vi "Gray's Mod Motor Controler.vi"() -> ()   [LabVIEW 2009]
uses:
  <vilib>/eio/EIONode/EIONode.xnode
  <vilib>/rvi/eio/nirviEIOImplementation/nirviEIOImplementation.xnode
  <vilib>/rvi/eio/common/nirviEmuTemplateMethod_noerrors.vi
  <vilib>/rvi/eio/common/nirviEmuClasses.ctl
  <vilib>/Platform/TimedLoop/XDataNode/XDataNode.xnode
  <vilib>/Platform/TimedLoop/XDataNode/loadlvalarms.vi
  <vilib>/Platform/TimedLoop/XDataNode/timing_clust.ctl
  <vilib>/Platform/TimedLoop/XDataNode/nitl_modes.ctl
  <vilib>/Platform/TimedLoop/XDataNode/wakeup.ctl
  <vilib>/Platform/TimedLoop/XDataNode/XDNodeRunTimeDep.lvlib
panel:
  in  "Steering Encoder Reset \nPosition Whole Rotations":i32
  in  "Counts per Drive Position 2":i32=205386
  in  "Drive Encoder Reset \nPosition Fractional":i32
  in  "Counts per Drive Position":i32=205386
  in  "Stop":bool=TRUE
  out "Drive Motor Speed (cpt)":fxp<+/-,20,1>
  out "Drive Encoder Delta (ticks)":u32
  in  "Drive Motor Speed Setpoint (mph)":fxp<+/-,20,7>
  in  "Drive Speed Proportional Control Feedback Gain":fxp<+/-,20,5>
  out "Drive Motor Speed (Volts)":fxp<+/-,20,5> format="%.17g"
  in  "Drive Conversion: \nmph to counts per tick":fxp<+/-,20,0>
  in  "Drive Encoder Offset":fxp<+/-,20,1>
  in  "Steering Proportional Control Feedback Gain":i32
  in  "Steer Motor Setpoint (degrees)":i8
  in  "Steering Encoder Offset from 0 counts":i32
  in  "Steering Conversion: degrees to ticks":i32
  out "Steering Motor Speed (Volts)":fxp<+/-,20,5> format="%.17g"
  out "Steering Position":i32
  out "Steering Encoder Index":i32
  out "Steering Encoder Raw":i32
  in  "Steering Encoder Reset":bool
  in  "Steering Encoder Reset \nPositions Fractional":i32
  out "Steering clock ticks/encoder count":u32
  in  "Drive Encoder Reset":bool
  in  "Drive Encoder Reset \nPosition Whole Rotations":i32
  out "Drive Encoder Index":i32
  out "Drive Position":i32
  # "Drive Motor Control"
  # "Steering Motor Control"
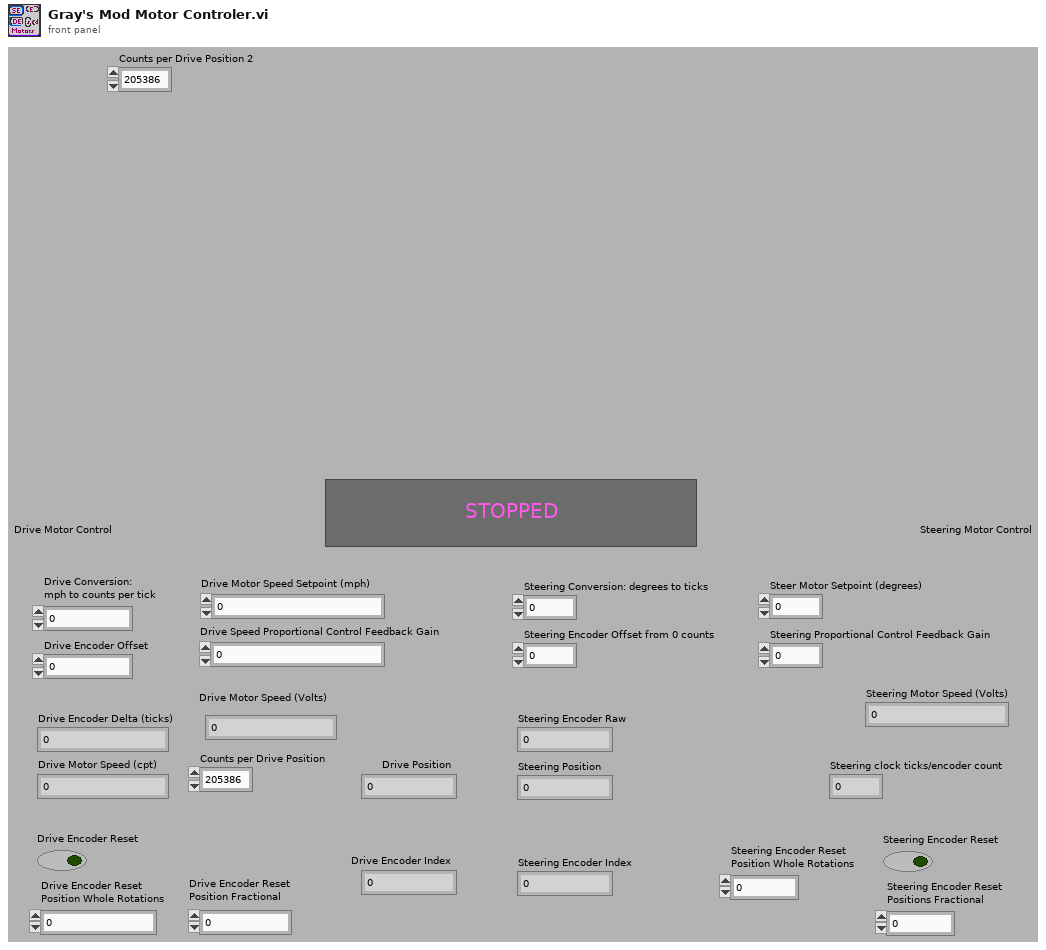
[diagram p1: front panel]
types:
  T1 = typedef "XDNodeRunTimeDep.lvlib/timing_clust.ctl" = cluster{"Expected End [f-1]":u64, "Actual End [f-1]":u64, "Finished Late? [f-1]":bool, "Expected End [i-1]":u64, "Actual End [i-1]":u64, "Finished Late? [i-1]":bool, "Expected Start [i]":u64, "Actual Start [i]":u64, "Expected Start [f]":u64, "Actual Start [f]":u64, "Source Name":string, "Structure Name":string, "Period":i64, "Deadline":i64, "Offset":i64, "Start":i64, "Priority":i32, "Timeout":i32, "Mode":T2, "Wakeup Reason":T3, "Error":errorcluster, "Source Type":string, "Secondary Source Type":string, "Global End Time":u64, "Global Start Time":u64, "Frame Duration":u64, "Iteration Duration":u64, "Assigned CPU":i32, "I/O Scan Engine Mode":u32}
  T2 = typedef "XDNodeRunTimeDep.lvlib/nitl_modes.ctl" = enum32{"No Change", "Process missed periods, maintain original phase", "Discard missed periods, maintain original phase", "Process missed periods, ignore original phase", "Discard missed periods, ignore original phase"}
  T3 = typedef "XDNodeRunTimeDep.lvlib/wakeup.ctl" = enum32{"Normal", "Aborted", "Asynchronous wakeup", "Timing source error", "Timed loop error", "Timeout"}
  T4 = typedef "nirviEmuClasses.ctl" = enum16{"IO Read", "IO Write", "Method", "Property Read", "Property Write"}
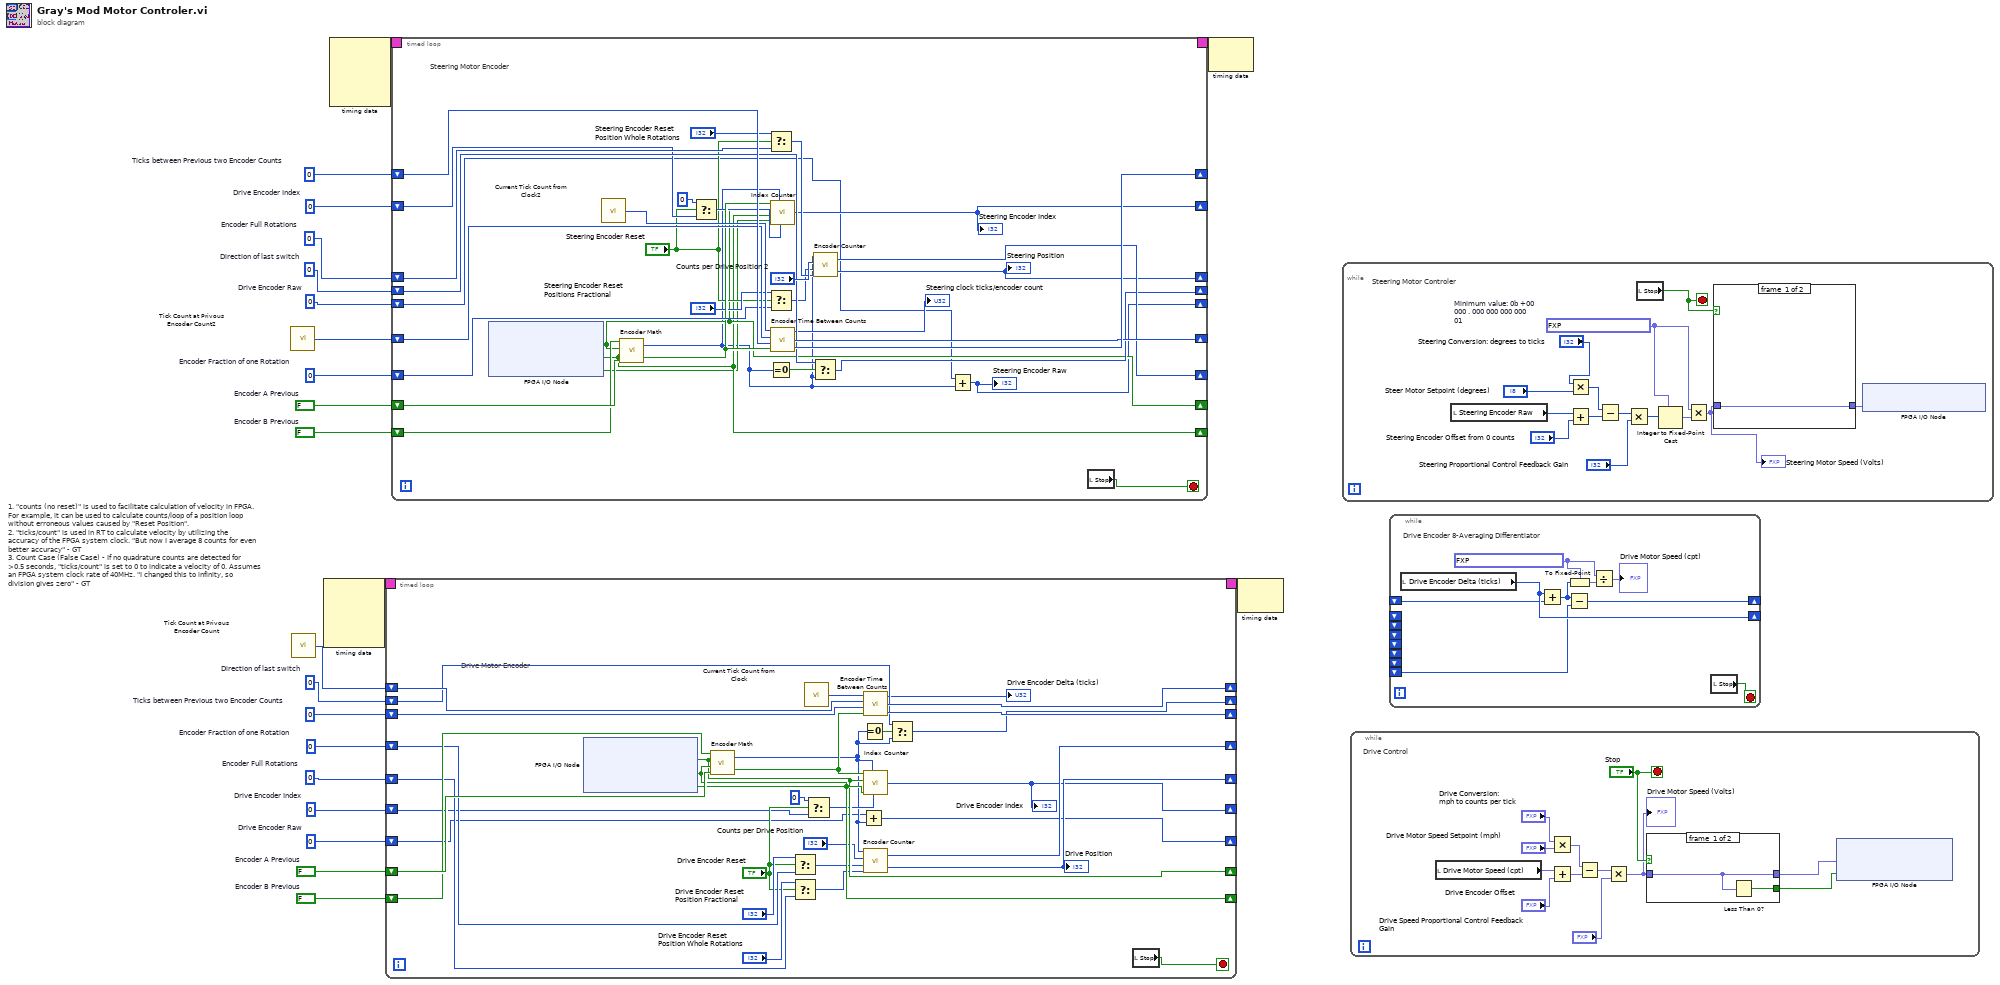
[diagram p0: block diagram]
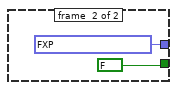
[diagram p2: hidden frame]
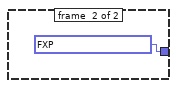
[diagram p3: hidden frame]
diagram:
  w9 = 0  # Direction of last switch
  w7 = FALSE  # Encoder B Previous
  w6 = FALSE  # Encoder A Previous
  w1 = 0  # Drive Encoder Raw
  w5 = u32 0  # Ticks between Previous two Encoder Counts
  w2 = 0  # Drive Encoder Index
  w4 = 0  # Encoder Fraction of one Rotation
  w3 = 0  # Encoder Full Rotations
  w12 = 0  # Direction of last switch
  w14 = FALSE  # Encoder B Previous
  w15 = FALSE  # Encoder A Previous
  w20 = 0  # Drive Encoder Raw
  w16 = u32 0  # Ticks between Previous two Encoder Counts
  w19 = 0  # Drive Encoder Index
  w17 = 0  # Encoder Fraction of one Rotation
  w18 = 0  # Encoder Full Rotations
  # "1. \"counts (no reset)\" is used to facilitate calculation of velocity in FPGA.\nFor example, it can be used to calculate counts/loop of a position loop\nwithout erroneous values caused by \"Reset Position\". \n2. \"ticks/count\" is used in RT to calculate velocity by utilizing the\naccuracy of the FPGA system clock. \"But now I average 8 counts for even\nbetter accuracy\" - GT\n3. Count Case (False Case) - If no quadrature counts are detected for\n>0.5 seconds, \"ticks/count\" is set to 0 to indicate a velocity of 0. Assumes\nan FPGA system clock rate of 40MHz. \"I changed this to infinity, so\ndivision gives zero\" - GT"
  n1 = call "Tick Count at Privous Encoder Count2"() -> ("Tick Count(Ticks)"=w8:u32)
  n2 = call "Tick Count at Privous Encoder Count"() -> ("Tick Count(Ticks)"=w13:u32)
  n3 = node-c288() -> (w22:T1)  [unwired: 4 in]
  n4 = node-c288() -> (w11:T1)  [unwired: 4 in]
  n5 = timed-loop {
    shift-right: [w51] -> _
    shift-left: w15 -> [w55]
    shift-right: [w53] -> _
    shift-left: w14 -> [w50]
    shift-right: [w30] -> _
    shift-left: w19 -> [w27]
    shift-right: [w45] -> _
    shift-left: w13 -> [w46]
    shift-right: [w48] -> _
    shift-left: w16 -> [w49]
    timing: w22 -> [_]
    timing-out: [_] -> w21
    shift-right: [w23] -> _
    shift-left: w20 -> [w24]
    shift-right: [w42] -> _
    shift-left: w18 -> [w37]
    shift-right: [w43] -> _
    shift-left: w17 -> [w33]
    shift-right: [w39] -> _
    shift-left: w12 -> [w40]
    stop <- w52 stop-if-true
    # "Drive Motor Encoder"
    n6 = xnode "FPGA I/O Node"() -> ("Drive Encoder A"=w51:bool, "Drive Encoder B"=w53:bool, "Drive Encoder Index"=w54:bool)  [unwired: 3 in, 3 out]
    n7 = call "Encoder Math.vi"("Encoder A_old"=w55, "Encoder B_old"=w53, "Encoder A_new"=w51, "Encoder B_new"=w50) -> ("The Encoder Changed"=w31:bool, "Change in Encoder Value"=w25:i32)
    n8 = Select(t="Drive Encoder Reset \nPosition Fractional", s="Drive Encoder Reset", f=w33) -> (s? t:f=w32:i32)
    n9 = Select(t="Drive Encoder Reset \nPosition Whole Rotations", s="Drive Encoder Reset", f=w37) -> (s? t:f=w36:i32)
    n10 = call "Current Tick Count from Clock"() -> ("Tick Count(Ticks)"=w47:u32)
    n11 = Select(t=0, s="Drive Encoder Reset", f=w27) -> (s? t:f=w26:i32)
    n12 = Add(x=w24, y=w25) -> (x+y=w23:i32)
    n13 = Equal To 0?(x=w25) -> (x = 0?=w41:bool)
    n14 = call "Encoder Time Between Counts.vi"("The Encoder Changed"=w31, "Ticks between Previous two Encoder Counts (n-1)"=w49, "Tick Count at Previous Encoder Count (n-1)"=w46, "Current Tick Count"=w47) -> ("Ticks between Previous two Encoder Counts (n)"=w48:u32, "Tick Count at Previous Encoder Count (n)"=w45:u32, "Encoder Delta (ticks)"=→"Drive Encoder Delta (ticks)":u32)
    n15 = call "Index Counter.vi"("Encoder Index (n-1)"=w26, "Change in Encoder Value"=w25, "Encoder Index Pin"=w54, "Encoder B Pin"=w53, "Encoder A Pin"=w51, "The Encoder Changed"=w31) -> ("Encoder Index (n)"=w30:i32)
    "Drive Encoder Index" <- w30
    n16 = call "Encoder Counter.vi"("Encoder Full Rotations (n-1)"=w36, "Encoder Fraction of one Rotation (n-1)"=w32, "Counts per Rotation"="Counts per Drive Position", "Change in Encoder Value"=w25) -> ("Encoder Full Rotations (n)"=w42:i32, "Encoder Fraction of one Rotation (n)"=w43:i32)
    "Drive Position" <- w42
    n17 = Select(t=w40, s=w41, f=w25) -> (s? t:f=w39:i32)
    n18 = local read "Stop"() -> (w52:bool)
  }
  n19 = timed-loop {
    shift-right: [w120] -> _
    shift-left: w6 -> [w147]
    shift-right: [w119] -> _
    shift-left: w7 -> [w145]
    shift-right: [w121] -> _
    shift-left: w2 -> [w128]
    shift-right: [w140] -> _
    shift-left: w8 -> [w141]
    shift-right: [w143] -> _
    shift-left: w5 -> [w144]
    timing: w11 -> [_]
    timing-out: [_] -> w10
    shift-right: [w115] -> _
    shift-left: w1 -> [w116]
    shift-right: [w122] -> _
    shift-left: w3 -> [w134]
    shift-right: [w138] -> _
    shift-left: w4 -> [w132]
    shift-right: [w135] -> _
    shift-left: w9 -> [w136]
    stop <- w146 stop-if-true
    # "Steering Motor Encoder"
    n20 = xnode "FPGA I/O Node"() -> ("Drive Encoder A"=w120:bool, "Drive Encoder B"=w119:bool, "Drive Encoder Index"=w118:bool)  [unwired: 3 in, 3 out]
    n21 = call "Current Tick Count from Clock2"() -> ("Tick Count(Ticks)"=w142:u32)
    n22 = call "Encoder Math.vi"("Encoder A_old"=w147, "Encoder B_old"=w119, "Encoder A_new"=w120, "Encoder B_new"=w145) -> ("The Encoder Changed"=w130:bool, "Change in Encoder Value"=w117:i32)
    n23 = Select(t=0, s="Steering Encoder Reset", f=w128) -> (s? t:f=w127:i32)
    n24 = Select(t="Steering Encoder Reset \nPosition Whole Rotations", s="Steering Encoder Reset", f=w134) -> (s? t:f=w133:i32)
    n25 = Select(t="Steering Encoder Reset \nPositions Fractional", s="Steering Encoder Reset", f=w132) -> (s? t:f=w131:i32)
    n26 = Equal To 0?(x=w117) -> (x = 0?=w137:bool)
    n27 = call "Index Counter.vi"("Encoder Index (n-1)"=w127, "Change in Encoder Value"=w117, "Encoder Index Pin"=w118, "Encoder B Pin"=w119, "Encoder A Pin"=w120, "The Encoder Changed"=w130) -> ("Encoder Index (n)"=w121:i32)
    "Steering Encoder Index" <- w121
    n28 = call "Encoder Time Between Counts.vi"("The Encoder Changed"=w130, "Ticks between Previous two Encoder Counts (n-1)"=w144, "Tick Count at Previous Encoder Count (n-1)"=w141, "Current Tick Count"=w142) -> ("Ticks between Previous two Encoder Counts (n)"=w143:u32, "Tick Count at Previous Encoder Count (n)"=w140:u32, "Encoder Delta (ticks)"=→"Steering clock ticks/encoder count":u32)
    n29 = Select(t=w136, s=w137, f=w117) -> (s? t:f=w135:i32)
    n30 = call "Encoder Counter.vi"("Encoder Full Rotations (n-1)"=w133, "Encoder Fraction of one Rotation (n-1)"=w131, "Counts per Rotation"="Counts per Drive Position 2", "Change in Encoder Value"=w117) -> ("Encoder Full Rotations (n)"=w122:i32, "Encoder Fraction of one Rotation (n)"=w138:i32)
    "Steering Position" <- w122
    n31 = Add(x=w116, y=w117) -> (x+y=w115:i32)
    "Steering Encoder Raw" <- w115
    n32 = local read "Stop"() -> (w146:bool)
  }
  n33 = node-c288(w10) -> ()  [unwired: 1 out]
  n34 = node-c288(w21) -> ()  [unwired: 1 out]
  n35 = while {
    stop <- w213 stop-if-true
    w218 = fxp<+/-,20,5> 3.0517578125e-05  # Minimum value: 0b +00 000 . 000 000 000 000 01
    # "Steering Motor Controler"
    n36 = local read "Steering Encoder Raw"() -> (w207:i32)
    n37 = Multiply(x="Steering Conversion: degrees to ticks", y="Steer Motor Setpoint (degrees)") -> (x*y=w217:i32)
    n38 = Add(x=w207, y="Steering Encoder Offset from 0 counts") -> (x+y=w216:i32)
    n39 = Subtract(x=w217, y=w216) -> (x-y=w220:i32)
    n40 = Multiply(x=w220, y="Steering Proportional Control Feedback Gain") -> (x*y=w215:i32)
    n41 = local read "Stop"() -> (w213:bool)
    n42 = Integer to Fixed-Point Cast(fixed-point type=w218, integer=w215) -> (fixed-point=w219:fxp<+/-,20,5>)
    n43 = Multiply(x=w218, y=w219) -> (x*y=w212:fxp<+/-,20,5>)
    "Steering Motor Speed (Volts)" <- w212
    n44 = case shown="False" w213 {
      tunnel: w212 -> [w221 _]
      tunnel: [w221 fxp<+/-,20,5> 0.0] -> w214
      frame #0 {
      }
      frame #1 {
      }
    }
    n45 = xnode "FPGA I/O Node"("Steering Motor Speed"=w214) -> ()  [unwired: 1 in, 1 out]
  }
  n46 = while {
    stop <- "Stop" stop-if-true
    # "Drive Control"
    n47 = local read "Drive Motor Speed (cpt)"() -> (w243:fxp<+/-,20,1>)
    n48 = Multiply(x="Drive Conversion: \nmph to counts per tick", y="Drive Motor Speed Setpoint (mph)") -> (x*y=w244:fxp<+/-,20,5>)
    n49 = Add(x=w243, y="Drive Encoder Offset") -> (x+y=w242:fxp<+/-,20,5>)
    n50 = Subtract(x=w244, y=w242) -> (x-y=w245:fxp<+/-,20,5>)
    n51 = Multiply(x=w245, y="Drive Speed Proportional Control Feedback Gain") -> (x*y=w235:fxp<+/-,20,5>)
    "Drive Motor Speed (Volts)" <- w235
    n52 = case shown="True" "Stop" {
      tunnel: w235 -> [w269 _]
      tunnel: [w269 fxp<+/-,20,5> 0.0] -> w241
      tunnel: [w268 FALSE] -> w234
      frame #0 {
        n53 = Less Than 0?(x=w269) -> (x < 0?=w268:bool)
      }
      frame #1 {
      }
    }
    n54 = xnode "FPGA I/O Node"("Drive Motor Speed"=w241, "Drive Motor Reverse"=w234) -> ()  [unwired: 2 in, 2 out]
  }
  n55 = while {
    shift-right: [w275] -> _
    shift-left: _ -> [w274]
    shift-right: [w277] -> _
    shift-left: _ -> [_]
    shift-left: _ -> [_]
    shift-left: _ -> [_]
    shift-left: _ -> [_]
    shift-left: _ -> [_]
    shift-left: _ -> [_]
    shift-left: _ -> [w273]
    stop <- w278 stop-if-true
    w279 = fxp<+/-,32,32> 8.0 ("fixed-point type")
    # "Drive Encoder 8-Averaging Differentiator"
    n56 = local read "Drive Encoder Delta (ticks)"() -> (w277:u32)
    n57 = Add(x=w277, y=w274) -> (x+y=w276:u32)
    n58 = Subtract(x=w276, y=w273) -> (x-y=w275:u32)
    n59 = To Fixed-Point(fixed-point type=w279, number=w276) -> (fixed-point=w280:fxp<+/-,32,32>)
    n60 = Divide(x=w279, y=w280) -> (x/y=→"Drive Motor Speed (cpt)":fxp<+/-,20,1>)
    n61 = local read "Stop"() -> (w278:bool)
  }
